vi "Optimiser Mode Panel.vi"(8 "error in (no error)":errorcluster, 11 "Optimiser SBlock in":refnum<class "Optimiser SBlock.lvclass">) -> (0 "error out":errorcluster, 2 "No. of exploration RUNs out":u32, 3 "Optimiser SBlock out":refnum<class "Optimiser SBlock.lvclass">)   [LabVIEW 2020, in "TALOS.lvlib" / "Run Utilities.lvlib" / "Optimiser SBlock.lvclass"]
uses:
  Optimiser SBlock.lvclass
  Optimiser Cell/Optimise parameter - numeric.ctl
  Optimiser Cell/Optimisation observable.ctl
  Optimiser Cell/Optimisation Strategy.ctl
  Optimiser Cell/Optimise parameter - string.ctl
  6ef89b25-175a-42bf-9e1f-a1fea358bbfc.vi
  <vilib>/Comparison/Equal/Equal Functor/Equal Functor.lvclass
  Optimiser Cell/Optimiser Cell.lvclass
panel:
  in  "Array from List":T1[](array[typedef])
  in  "Array of Observables":T2[](array[typedef]) caption="Observable name                                                                  Weight" {"Weight" min=0.0 max=1.0}
  in  "Array of Parameters":T3[](array[typedef]) caption="Parameter"
  in  "Value":dbl
  in  "Strategy":T4
  in  "explorers":u16 caption="No. of exploration RUNs"
  # "Parameters - Numeric"
  # "Start value"
  # "From"
  # "To"
  # "dtype"
  # "Parameters - String"
  # "Start value"
  # "Available options"
  # "Observables"
  # "Weight"
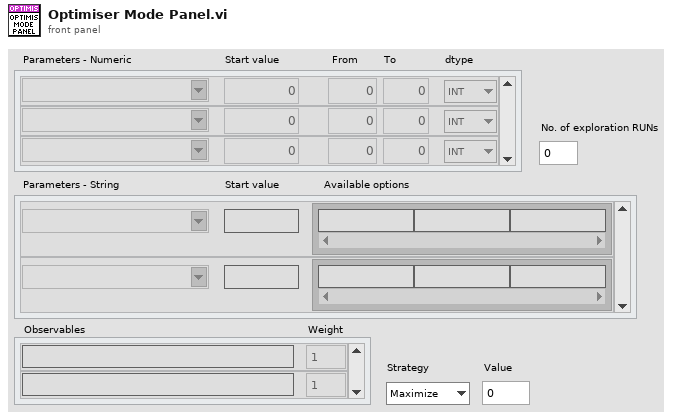
[diagram p1: front panel]
types:
  T1 = typedef "TALOS.lvlib/Run Utilities.lvlib/Optimiser Cell.lvclass/Optimise parameter - string.ctl" = cluster{"Name":string, "Start value":string, "Options":string[]}
  T2 = typedef "TALOS.lvlib/Run Utilities.lvlib/Optimiser Cell.lvclass/Optimisation observable.ctl" = cluster{"Name":string, "Weight":dbl}
  T3 = typedef "TALOS.lvlib/Run Utilities.lvlib/Optimiser Cell.lvclass/Optimise parameter - numeric.ctl" = cluster{"Name":string, "Start value":dbl, "From":dbl, "To":dbl, "dtype":enum16{"INT", "DBL"}}
  T4 = typedef "TALOS.lvlib/Run Utilities.lvlib/Optimiser Cell.lvclass/Optimisation Strategy.ctl" = enum16{"Maximize", "Minimize", "Value"}
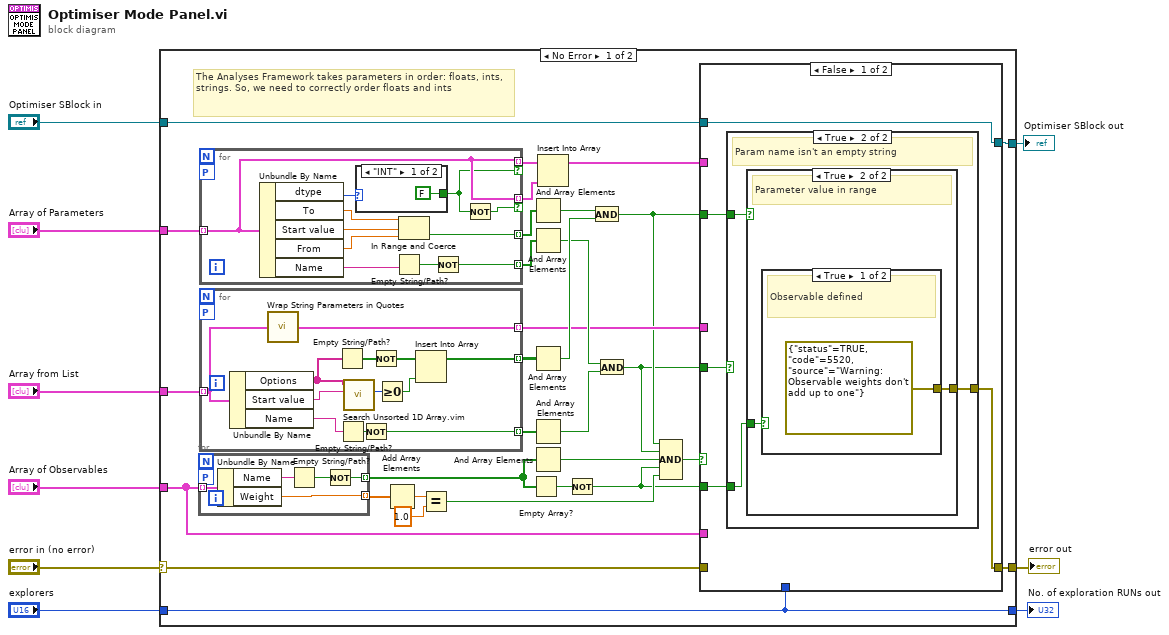
[diagram p0: block diagram]
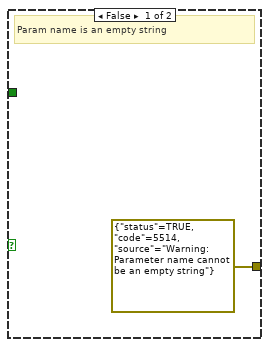
[diagram p2: hidden frame]
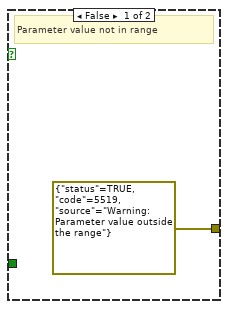
[diagram p3: hidden frame]
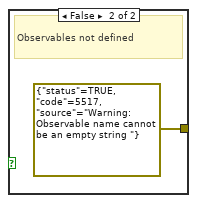
[diagram p4: hidden frame]
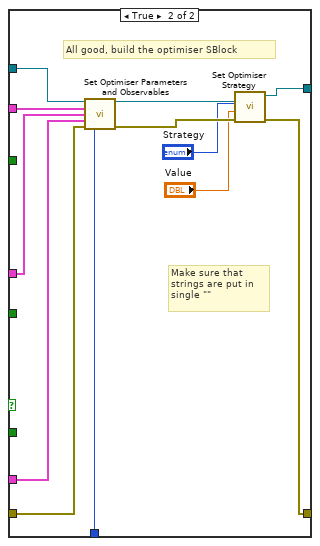
[diagram p5: hidden frame]
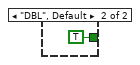
[diagram p6: hidden frame]
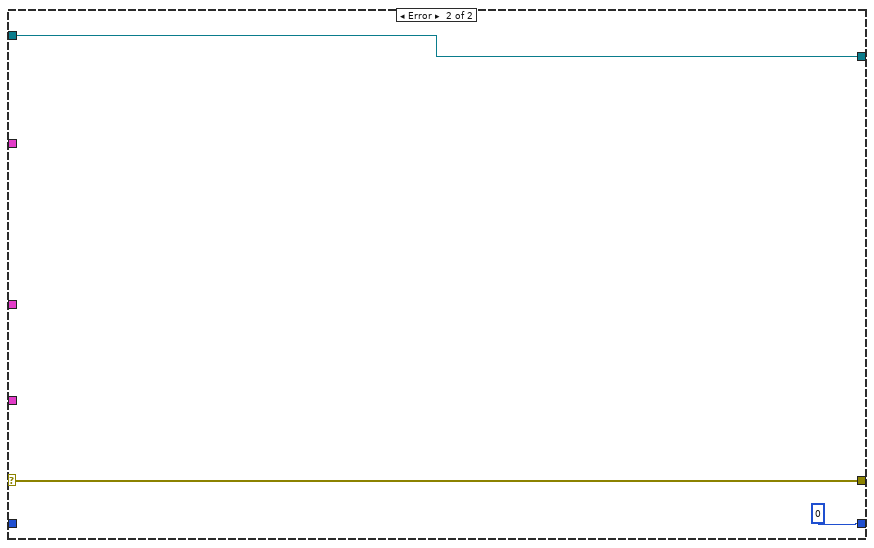
[diagram p7: hidden frame]
diagram:
  n1 = case shown="No Error" "error in (no error)" {
    selector: "error in (no error)" -> [w36 w98]
    tunnel: "Optimiser SBlock in" -> [w39 w97]
    tunnel: [w38 w97] -> w8
    tunnel: "Array of Parameters" -> [w34 _]
    tunnel: "Array of Observables" -> [w14 _]
    tunnel: [w37 w98] -> w5
    tunnel: "explorers" -> [w35 _]
    tunnel: [w35 u32 0 ("No. of exploration RUNs")] -> w2
    tunnel: "Array from List" -> [w20 _]
    frame No Error {
      # "The Analyses Framework takes parameters in order: floats, ints, strings. So, we need to correctly order floats and ints"
      n2 = for {
        tunnel: w14 -> [w57] mode=indexing
        tunnel: [w53] -> w30 mode=indexing
        tunnel: [w54] -> w28 mode=indexing
        workers-P: _ -> [_]
        n3 = Unbundle By Name(w57) -> ("Name"=w56:string, "Weight"=w54:dbl)
        n4 = Empty String/Path?(string/path=w56) -> (empty?=w55:bool)
        n5 = Not(x=w55) -> (.not. x?=w53:bool)
      }
      n6 = for {
        tunnel: w34 -> [w86] mode=indexing
        tunnel: [w92] -> w33 mode=indexing
        tunnel: [w88] -> w32 mode=indexing
        tunnel: [w86] -> w18 mode=indexing if=w85
        tunnel: [w86] -> w17 mode=indexing if=w84
        workers-P: _ -> [_]
        n7 = Unbundle By Name(w86) -> ("dtype"=w87:enum16{"INT", "DBL"}, "To"=w91:dbl, "Start value"=w89:dbl, "From"=w90:dbl, "Name"=w94:string)
        n8 = case shown="\"INT\"" w87 {
          tunnel: [FALSE TRUE] -> w85
          frame "INT" {
          }
          frame "DBL", Default {
          }
        }
        n9 = Empty String/Path?(string/path=w94) -> (empty?=w93:bool)
        n10 = In Range and Coerce(upper limit=w91, x=w89, lower limit=w90) -> (In Range?=w88:bool)  [unwired: 1 out]
        n11 = Not(x=w93) -> (.not. x?=w92:bool)
        n12 = Not(x=w85) -> (.not. x?=w84:bool)
      }
      n13 = for {
        tunnel: [w51] -> w23 mode=indexing
        tunnel: w20 -> [w42] mode=indexing
        tunnel: [w47] -> w22 mode=indexing
        tunnel: [w41] -> w19 mode=indexing
        workers-P: _ -> [_]
        n14 = Unbundle By Name(w42) -> ("Options"=w44:string[], "Start value"=w43:string, "Name"=w45:string)
        n15 = call "Wrap String Parameters in Quotes.vi"("Optimise parameter - string in"=w42) -> ("Optimise parameter - string out"=w41:T1)
        n16 = Empty String/Path?(string/path=w44) -> (empty?=w50:bool[])
        n17 = Empty String/Path?(string/path=w45) -> (empty?=w52:bool)
        n18 = call "Search Unsorted 1D Array.vim"("element"=w43, "unsorted 1D array"=w44) -> ("index of element"=w49:i32)  [unwired: 9 in]
        n19 = Not(x=w52) -> (.not. x?=w51:bool)
        n20 = Not(x=w50) -> (.not. x?=w46:bool[])
        n21 = Greater Or Equal To 0?(x=w49) -> (x >= 0?=w48:bool)
        n22 = Insert Into Array(array=w46, new element=w48) -> (w47:bool[])  [unwired: 1 in]
      }
      n23 = Add Array Elements(numeric array=w28) -> (sum=w27:dbl)
      n24 = Equal?(x=w27, y=1.0) -> (x = y?=w11:bool)
      n25 = Empty Array?(array=w30) -> (empty?=w29:bool)
      n26 = And Array Elements(Boolean array=w32) -> (logical AND=w21:bool)
      n27 = And Array Elements(Boolean array=w33) -> (logical AND=w24:bool)
      n28 = And Array Elements(Boolean array=w22) -> (logical AND=w40:bool)
      n29 = And Array Elements(Boolean array=w23) -> (logical AND=w25:bool)
      n30 = And Array Elements(Boolean array=w30) -> (logical AND=w31:bool)
      n31 = Insert Into Array(array=w18, new element=w17) -> (w16:T3[])  [unwired: 1 in]
      n32 = Not(x=w29) -> (.not. x?=w10:bool)
      n33 = And(x=w21, y=w40) -> (x .and. y?=w15:bool)
      n34 = And(x=w24, y=w25) -> (x .and. y?=w12:bool)
      n35 = Compound Arithmetic op=AND(w15, w12, w31, w10, w11) -> (w13:bool)
      n36 = case shown="False" w13 {
        tunnel: w39 -> [w62 w80]
        tunnel: [w62 w76] -> w38
        tunnel: w16 -> [_ w83]
        tunnel: w14 -> [_ w82]
        tunnel: w35 -> [_ w73]
        tunnel: [w61 w75] -> w37
        tunnel: w36 -> [_ w81]
        tunnel: w19 -> [_ w72]
        tunnel: w15 -> [w59 _]
        tunnel: w12 -> [w60 _]
        tunnel: w10 -> [w58 _]
        frame False {
          n37 = case shown="True" w60 {
            tunnel: [errorcluster {"status"=TRUE, "code"=5514, "source"="Warning: Parameter name cannot be an empty string"} ("error out") w66] -> w61
            tunnel: w59 -> [_ w65]
            tunnel: w58 -> [_ w64]
            frame False {
              # "Param name is an empty string"
            }
            frame True {
              # "Param name isn't an empty string"
              n38 = case shown="True" w65 {
                tunnel: [errorcluster {"status"=TRUE, "code"=5519, "source"="Warning: Parameter value outside the range"} ("error out") w69] -> w66
                tunnel: w64 -> [_ w68]
                frame False {
                  # "Parameter value not in range"
                }
                frame True {
                  # "Parameter value in range"
                  n39 = case shown="True" w68 {
                    tunnel: [errorcluster {"status"=TRUE, "code"=5520, "source"="Warning: Observable weights don't add up to one"} ("error out") errorcluster {"status"=TRUE, "code"=5517, "source"="Warning: Observable name cannot be an empty string "} ("error out")] -> w69
                    frame True {
                      # "Observable defined"
                    }
                    frame False {
                      # "Observables not defined"
                    }
                  }
                }
              }
            }
          }
        }
        frame True {
          # "Make sure that strings are put in single \"\""
          # "All good, build the optimiser SBlock"
          n40 = call-dynamic "Set Optimiser Parameters and Observables.vi"("Optimiser SBlock in"=w80, "Parameters"=w83, "Parameters - string"=w72, "Observables"=w82, "error in (no error)"=w81, "Number of Exploration Runs"=w73) -> ("Optimiser SBlock out"=w79:refnum<class "Optimiser SBlock.lvclass">, "error out"=w78:errorcluster)  [unwired: 8 in]
          n41 = call-dynamic "Set Optimiser Strategy.vi"("error in (no error)"=w78, "Value"="Value", "Optimisation method"="Strategy", "Optimiser SBlock in"=w79) -> ("error out"=w75:errorcluster, "Optimiser SBlock out"=w76:refnum<class "Optimiser SBlock.lvclass">)  [unwired: 6 in]
        }
      }
    }
    frame Error {
    }
  }
  "error out" <- w5
  "No. of exploration RUNs out" <- w2
  "Optimiser SBlock out" <- w8
